vi "calc_C_clarified.vi"(1 "H_FILTER":dbl, 2 "floc_sat":dbl, 3 "C_floc":dbl, 4 "C_coag":dbl, 5 "C_raw":dbl, 6 "kc":dbl) -> (0 "calc_C_clarified":dbl)   [LabVIEW 2019]
panel:
  # "Inputs"
  # "Outputs"
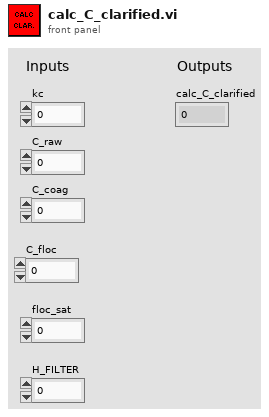
[diagram p1: front panel]
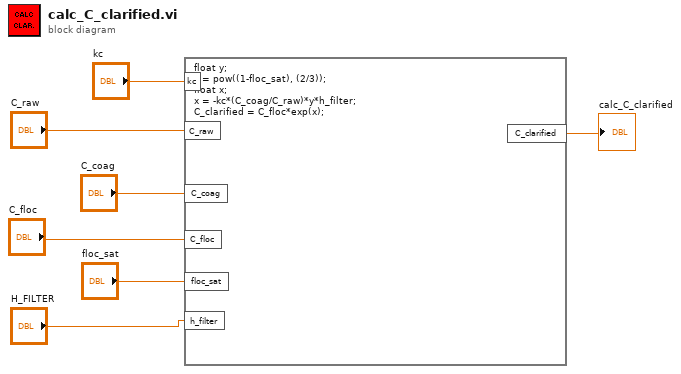
[diagram p0: block diagram]
diagram:
  n1 = formula code="float y;\ny = pow((1-floc_sat), (2/3));\nfloat x;\nx = -kc*(C_coag/C_raw)*y*h_filter;\nC_clarified = C_floc*exp(x);"("kc"="kc", "C_raw"="C_raw", "C_coag"="C_coag", "C_floc"="C_floc", "floc_sat"="floc_sat", "h_filter"="H_FILTER") -> ("C_clarified"=→"calc_C_clarified":dbl)
